vi "SendCmdNormal.vi"(8 "error in (no error)":errorcluster, 10 "index":i32, 11 "DataIn":string) -> (0 "error out":errorcluster, 2 "TimeOut":bool, 3 "Reccmd":string)   [LabVIEW 2019]
uses:
  LLB/Commonly VI.lvlib
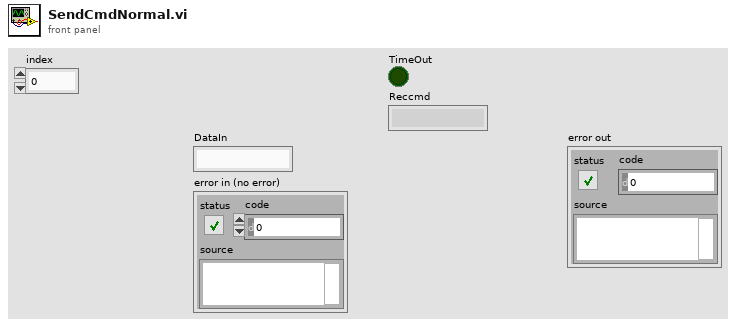
[diagram p1: front panel]
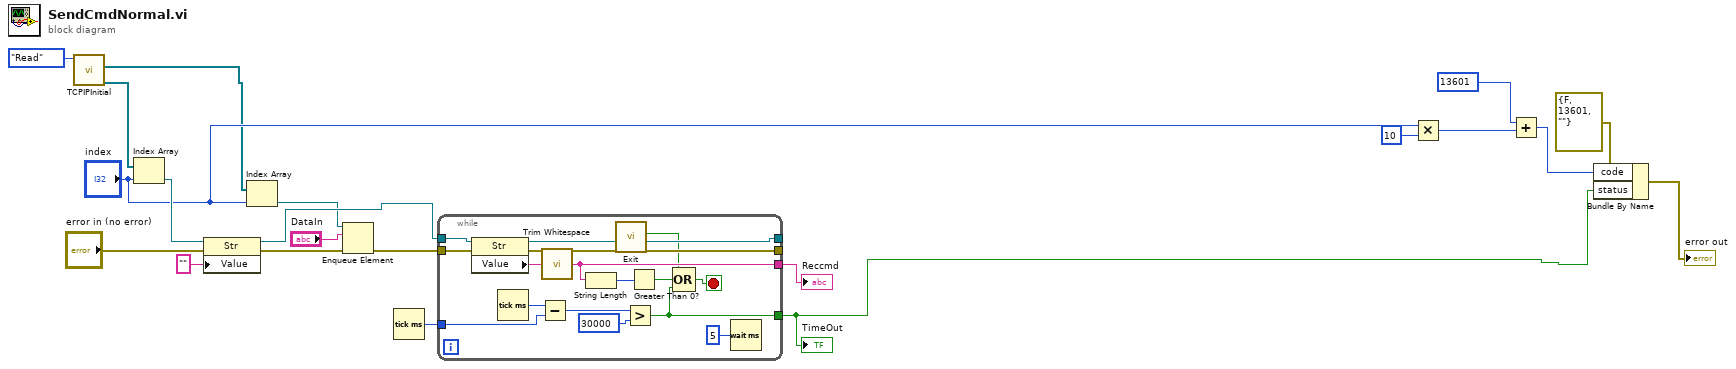
[diagram p0: block diagram]
diagram:
  n1 = call "TCPIPInitial.vi"("Enum"=enum16{"initial", "Read", "release"}."Read") -> ("SN_ReplyRef"=w2:refnum<vi>[], "Sn_cmdQ"=w3:refnum<queue>[])  [unwired: 7 in, 2 out]
  n2 = Index Array(array=w2, index="index") -> (element=w13:refnum<vi>)
  n3 = property class="Str"(reference=w13, error in="error in (no error)", "Value"="") -> (reference out=w17:refnum<vi>, error out=w19:errorcluster)
  n4 = Index Array(array=w3, index="index") -> (element=w12:refnum<queue>)
  n5 = Enqueue Element(queue=w12, element="DataIn", error in (no error)=w19) -> (error out=w15:errorcluster)  [unwired: 1 in, 2 out]
  n6 = Tick Count (ms)() -> (millisecond timer value=w16:u32)
  n7 = while {
    tunnel: w17 -> [w36]
    tunnel: w16 -> [w34]
    tunnel: w15 -> [w28]
    tunnel: [w27] -> _
    tunnel: [w26] -> w1
    tunnel: [w25] -> w14
    tunnel: [w23] -> _
    stop <- w29 stop-if-true
    n8 = property class="Str"(reference=w36, error in=w28) -> (reference out=w23:refnum<vi>, error out=w27:errorcluster, "Value"=w37:string)
    n9 = Tick Count (ms)() -> (millisecond timer value=w33:u32)
    n10 = Subtract(x=w33, y=w34) -> (x-y=w32:u32)
    n11 = call <vilib>:"Trim Whitespace.vi"("string"=w37) -> ("trimmed string"=w25:string)  [unwired: 1 in]
    n12 = String Length(string=w25) -> (length=w35:i32)
    n13 = call "Exit.vi"() -> ("ExitOut"=w22:bool)  [unwired: 11 in]
    n14 = Greater?(x=w32, y=u32 30000) -> (0:w26:bool)
    n15 = Greater Than 0?(x=w35) -> (x > 0?=w30:bool)
    n16 = Compound Arithmetic op=OR(w22, w30, w26) -> (w29:bool)
    n17 = Wait (ms)(milliseconds to wait=u32 5 ("millisecond timer value")) -> ()  [unwired: 1 out]
  }
  "TimeOut" <- w1
  "Reccmd" <- w14
  n18 = Multiply(x="index", y=10) -> (x*y=w5:i32)
  n19 = Add(x=13601 ("code"), y=w5) -> (x+y=w9:i32)
  n20 = Bundle By Name(cluster=errorcluster {"status"=FALSE, "code"=13601, "source"=""} ("error constant"), "code"=w9, "status"=w1) -> (→"error out":errorcluster)
